vi "7 Segment MC.vi"(1 "se":bool, 5 "sa":bool, 7 "sb":bool, 9 "sc":bool, 11 "sd":bool, 12 "sf":bool) -> (0 "a":bool)   [LabVIEW 2012]
panel:
  in  "sdp":bool
  in  "sg":bool
  out "dp":bool
  out "e":bool
  out "f":bool
  out "c":bool
  out "d":bool
  out "g":bool
  out "b":bool
  # "Run Continuously"
  # "0"
  # "7 Segment Display"
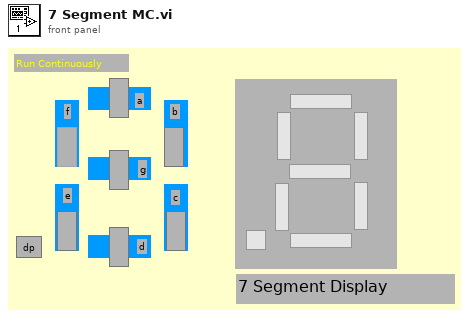
[diagram p1: front panel]
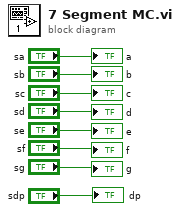
[diagram p0: block diagram]
diagram:
  "a" <- "sa"
  "b" <- "sb"
  "g" <- "sg"
  "d" <- "sd"
  "c" <- "sc"
  "f" <- "sf"
  "e" <- "se"
  "dp" <- "sdp"
